vi "读取Request Events.vi"(8 "error in (no error)":errorcluster caption="错误输入（无错误）", 11 "WebDAV client输入":refnum<class "WebDAV client.lvclass">) -> (0 "error out":errorcluster caption="错误输出", 2 "Request Events":refnum<event-registration> caption="请求事件", 3 "WebDAV client输出":refnum<class "WebDAV client.lvclass">)   [LabVIEW 2016, in "数据传输系统.lvlib" / "update.lvlib" / "WebDAV client.lvclass"]
uses:
  WebDAV client.lvclass
  <vilib>/WebDAVClient/Advanced/Multi Event/WebDAV Request Events.ctl
  <vilib>/WebDAVClient/Advanced/Multi Event/Request Progress.ctl
  <vilib>/WebDAVClient/Advanced/Multi Event/Asynchronous Session Handle.ctl
  <vilib>/WebDAVClient/Advanced/Multi Event/Asynchronous Request Handle.ctl
  <vilib>/WebDAVClient/Advanced/Multi Event/Request Complete.ctl
  <vilib>/WebDAVClient/Advanced/Multi Event/Request Status.ctl
  <vilib>/WebDAVClient/Advanced/Multi Event/List Directory Complete.ctl
  <vilib>/WebDAVClient/Advanced/FileInfo.ctl
  <vilib>/WebDAVClient/Advanced/Multi Event/Path Info Complete.ctl
  <vilib>/WebDAVClient/Advanced/Multi Event/Get Buffer Complete.ctl
  WebDAV client.lvclass/WebDAV client.ctl
  <vilib>/WebDAVClient/NI_WebDAV.lvlib
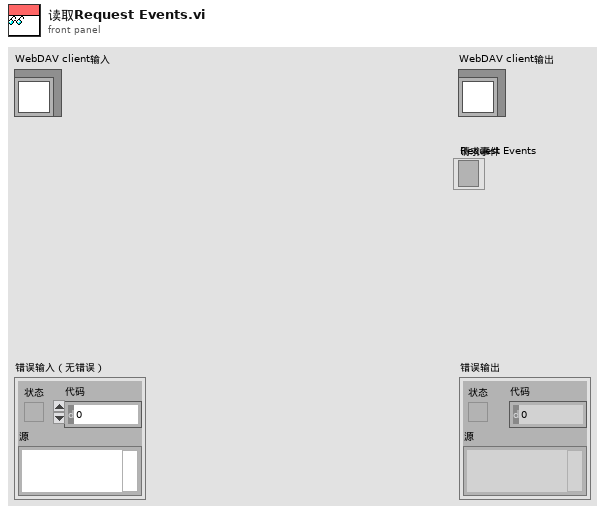
[diagram p1: front panel]
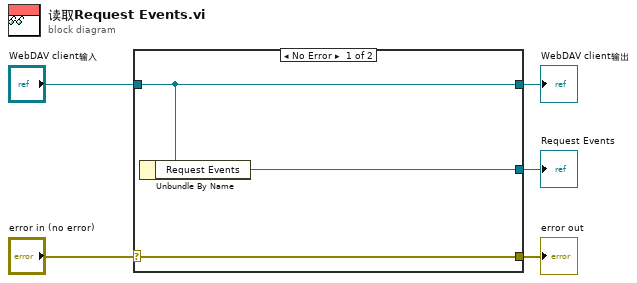
[diagram p0: block diagram]
diagram:
  n1 = case shown="No Error" "error in (no error)" {
    selector: "error in (no error)" -> [w8 w9]
    tunnel: [w8 w9] -> w4
    tunnel: [w7 w10] -> w2
    tunnel: "WebDAV client输入" -> [w7 w10]
    tunnel: [w6 _] -> w1
    frame No Error {
      n2 = Unbundle By Name(w7) -> ("Request Events"=w6:refnum<event-registration>)
    }
    frame Error {
    }
  }
  "error out" <- w4
  "WebDAV client输出" <- w2
  "Request Events" <- w1
